vi "to_perc.vi"() -> ()   [LabVIEW 2020]
uses:
  <vilib>/Utility/file.llb/Read Delimited Spreadsheet (DBL).vi
  <vilib>/Utility/file.llb/Write Delimited Spreadsheet (DBL).vi
  <vilib>/Analysis/NI_AALPro.lvlib
panel:
  out "data 2":dbl[][](array[numeric])
  out "Intensity Graph 2":dbl[][](graph)
  in  "Stop":i32
  in  "Start":i32
  out "Intensity Graph":dbl[][](graph)
  out "data":dbl[][](array[numeric])
  out "wavelength":dbl[](array[numeric])
  out "time delay":dbl[](array[numeric])
  in  "file path (dialog if empty)":path=path "C:/Users/Elyse/Desktop/Antoine/cut dat chirp correction/20200303-water-3P-AVERAGED-14-46-cut-chirp-correct.dat"
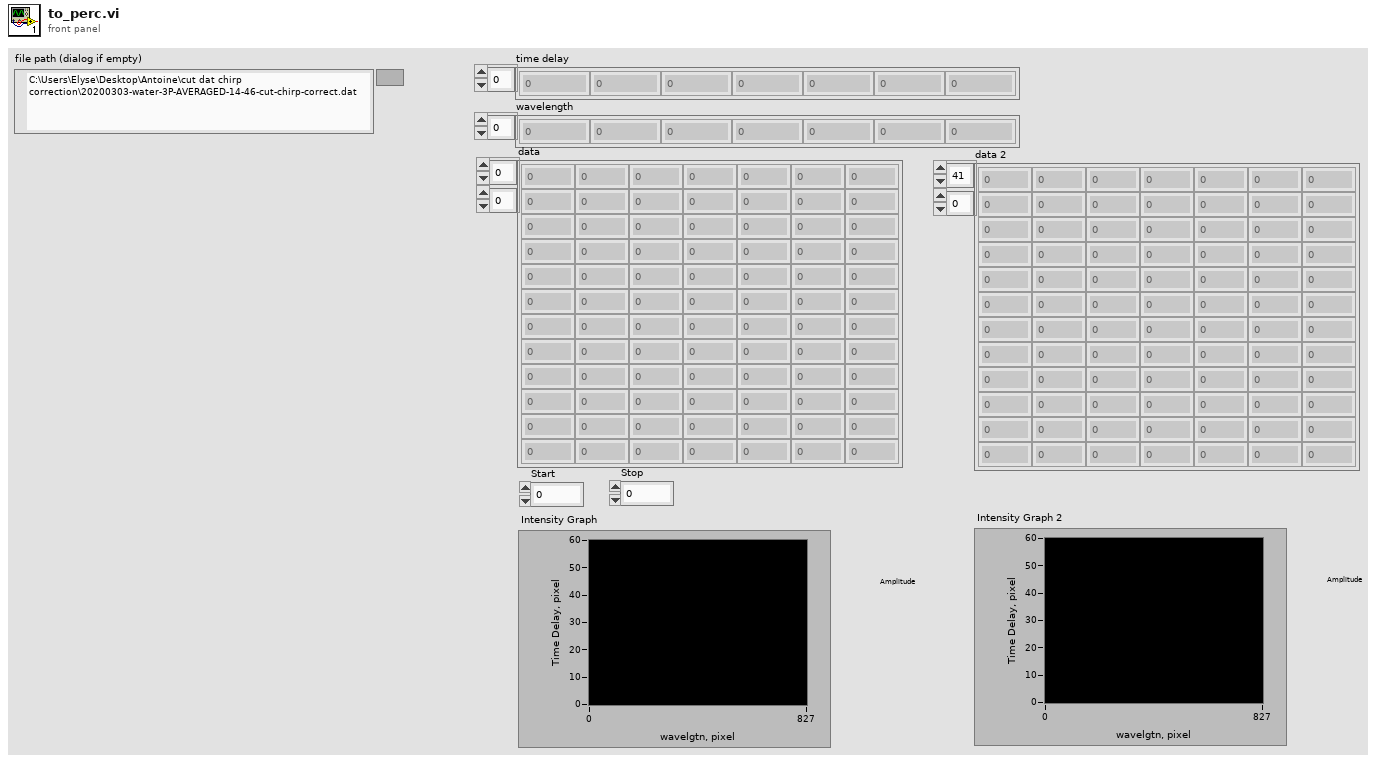
[diagram p1: front panel]
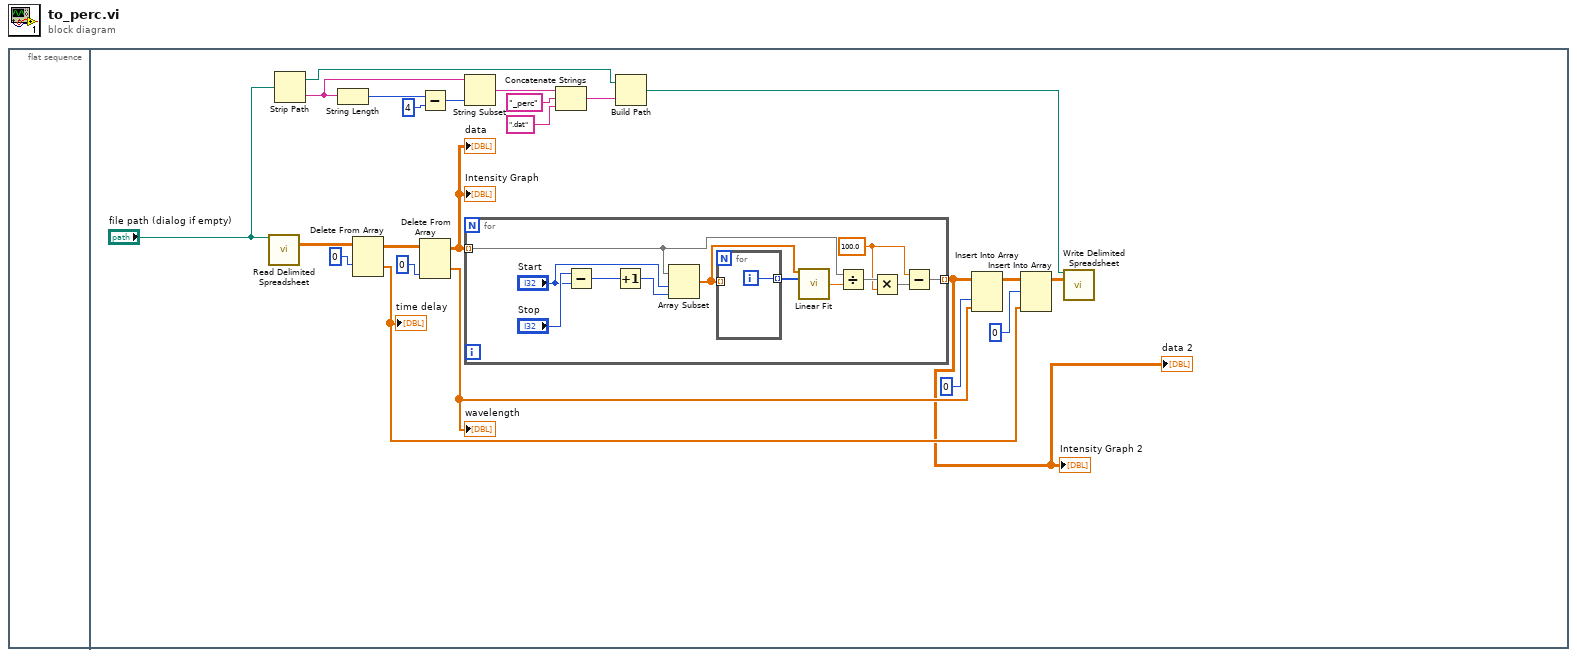
[diagram p0: block diagram]
diagram:
  n1 = flat-sequence {
    frame #0 {
    }
    frame #1 {
      n2 = call-poly <vilib>:"Read Delimited Spreadsheet.vi"("file path (dialog if empty)"="file path (dialog if empty)") -> ("all rows"=w20:dbl[][])  [unwired: 9 in, 5 out]
      n3 = Strip Path(path="file path (dialog if empty)") -> (stripped path=w4:path, name=w11:string)
      n4 = String Length(string=w11) -> (length=w10:i32)
      n5 = Delete From Array(array=w20, index (row)=0) -> (deleted portion=w15:dbl[], array with subset deleted=w22:dbl[][])  [unwired: 2 in]
      "time delay" <- w15
      n6 = Subtract(x=w10, y=4) -> (x-y=w8:i32)
      n7 = Delete From Array(array=w22, index (col)=0 ("disabled index (col)")) -> (deleted portion=w18:dbl[], array with subset deleted=w19:dbl[][])  [unwired: 2 in]
      "wavelength" <- w18
      "data" <- w19
      "Intensity Graph" <- w19
      n8 = String Subset(string=w11, length (rest)=w8) -> (substring=w7:string)  [unwired: 1 in]
      n9 = for {
        tunnel: w19 -> [w29] mode=indexing
        tunnel: [w24] -> w1 mode=indexing
        w26 = 100.0
        n10 = Subtract(x="Stop", y="Start") -> (x-y=w33:i32)
        n11 = Increment(x=w33) -> (x+1=w32:i32)
        n12 = Array Subset(array=w29, index="Start", length=w32) -> (w31:dbl[])
        n13 = for {
          tunnel: w31 -> [_] mode=indexing
          tunnel: [w36] -> w30 mode=indexing
          i -> [w36]
        }
        n14 = call <vilib>:"Linear Fit.vi"("Y"=w31, "X"=w30) -> ("intercept"=w28:dbl)  [unwired: 9 in, 4 out]
        n15 = Divide(x=w29, y=w28) -> (x/y=w27:dbl[])
        n16 = Multiply(x=w27, y=w26) -> (x*y=w25:dbl[])
        n17 = Subtract(x=w26, y=w25) -> (x-y=w24:dbl[])
      }
      "Intensity Graph 2" <- w1
      "data 2" <- w1
      n18 = Concatenate Strings(w7, "_perc" ("string"), ".dat" ("string")) -> (w3:string)
      n19 = Build Path(base path=w4, name or relative path=w3) -> (appended path=w2:path)
      n20 = Insert Into Array(array=w1, index (col)=0 ("disabled index (col)"), new element=w18) -> (w16:dbl[][])  [unwired: 1 in]
      n21 = Insert Into Array(array=w16, index (row)=0, new element=w15) -> (w13:dbl[][])  [unwired: 1 in]
      n22 = call-poly <vilib>:"Write Delimited Spreadsheet.vi"("file path (dialog if empty)"=w2, "2D data"=w13) -> ()  [unwired: 12 in, 2 out]
    }
  }
